vi "Enable Channel Save.vi"(8 "error in (no error)":errorcluster, 11 "Device Item Ref in":T1 format="%.0x") -> (0 "error out":errorcluster, 3 "Device Item Ref out":T1 format="%.0x")   [LabVIEW 2009, in "NI-XNET Custom Device.lvlib"]
doc: "This VI is automatically called when the channel configuration is saved. Look at the .xml file to see how to enable this VI to be called automatically."
uses:
  NI-XNET Custom Device.lvlib
  <vilib>/NI VeriStand/Custom Device API/Custom Device Item Ref.ctl
  <vilib>/NI VeriStand/Custom Device API/Set Item Property (String).vi
  <vilib>/NI VeriStand/Custom Device API/Get Item Property (Variant).vi
  <vilib>/NI VeriStand/Custom Device API/Custom Device API.lvlib
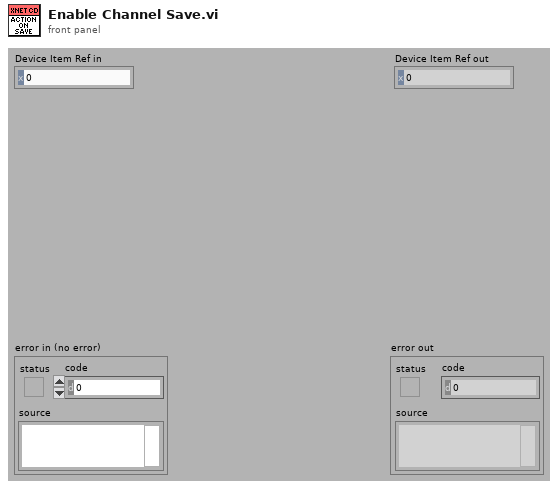
[diagram p1: front panel]
types:
  T1 = typedef "Custom Device API.lvlib/Custom Device Item Ref.ctl" = u64
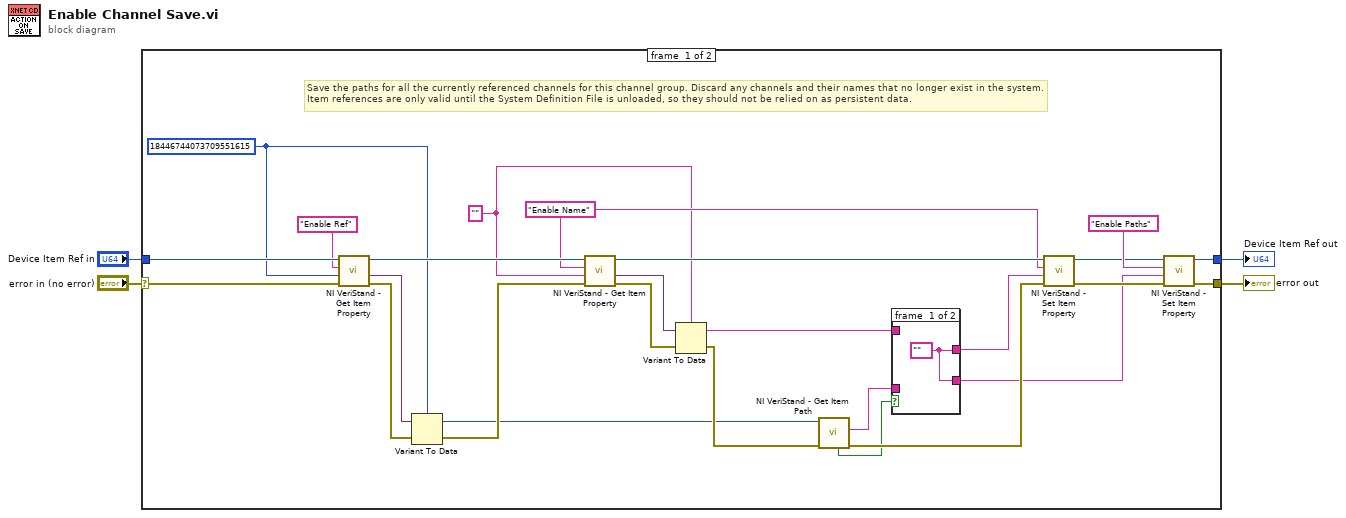
[diagram p0: block diagram]
diagram:
  n1 = case shown="No Error" "error in (no error)" {
    selector: "error in (no error)" -> [w26 w35]
    tunnel: [w20 w35] -> w3
    tunnel: "Device Item Ref in" -> [w25 w34]
    tunnel: [w19 w34] -> w1
    frame #0 {
      w7 = "" ("Path")
      w8 = "Enable Name" ("Property Name")
      w9 = T1 18446744073709551615 ("Device Item Ref in")
      # "Save the paths for all the currently referenced channels for this channel group. Discard any channels and their names that no longer exist in the system. Item references are only valid until the System Definition File is unloaded, so they should not be relied on as persistent data."
      n2 = call-poly <vilib>:"NI VeriStand - Get Item Property.vi"("error in (no error)"=w26, "Default Value"=w9, "Property Name"="Enable Ref", "Item Ref in"=w25) -> ("error out"=w23:errorcluster, "Value"=w22:variant, "Item Ref out"=w16:T1)  [unwired: 5 out]
      n3 = Variant To Data(error in=w23, Variant=w22, type=w9) -> (error out=w27:errorcluster, data=w18:T1)
      n4 = call-poly <vilib>:"NI VeriStand - Get Item Property.vi"("error in (no error)"=w27, "Default Value"=w7, "Property Name"=w8, "Item Ref in"=w16) -> ("error out"=w14:errorcluster, "Value"=w15:variant, "Item Ref out"=w12:T1)  [unwired: 5 out]
      n5 = Variant To Data(error in=w14, Variant=w15, type=w7) -> (error out=w28:errorcluster, data=w13:string)
      n6 = call <vilib>:"NI VeriStand - Get Item Path.vi"("error in (no error)"=w28, "Item Ref in"=w18) -> ("error out"=w30:errorcluster, "Path"=w5:string, "Found"=w6:bool)  [unwired: 7 out]
      n7 = case shown="True" w6 {
        tunnel: [w31 w32] -> w17
        tunnel: w5 -> [_ w32]
        tunnel: [w31 w33] -> w11
        tunnel: w13 -> [_ w33]
        frame #0 {
          w31 = "" ("Path")
        }
        frame #1 {
        }
      }
      n8 = call-poly <vilib>:"NI VeriStand - Set Item Property.vi"("error in (no error)"=w30, "Value"=w11, "Property Name"=w8, "Item Ref in"=w12) -> ("error out"=w29:errorcluster, "Item Ref out"=w10:T1)  [unwired: 6 out]
      n9 = call-poly <vilib>:"NI VeriStand - Set Item Property.vi"("error in (no error)"=w29, "Value"=w17, "Property Name"="Enable Paths", "Item Ref in"=w10) -> ("error out"=w20:errorcluster, "Item Ref out"=w19:T1)  [unwired: 6 out]
    }
    frame #1 {
    }
  }
  "error out" <- w3
  "Device Item Ref out" <- w1
